vi "Traverse_Space_Server.vi"(6 "Probe Support":T1=[{"Max"=15.0, "Min"=-15.0}, {"Max"=250.0, "Min"=0.0}, {"Max"=15.0, "Min"=-15.0}] {"Min" format="%#.1f"; "Max" format="%#.1f"}, 7 "Mode":T4(ring), 8 "Traverse Limits":T1=[{"Max"=15001.0, "Min"=12000.0}, {"Max"=1000.0, "Min"=-1000.0}, {"Max"=700.0, "Min"=0.0}] {"Min" format="%#.1f"; "Max" format="%#.1f"}, 9 "Probe Volume":T1=[{"Max"=0.0, "Min"=0.0}, {"Max"=250.0, "Min"=0.0}, {"Max"=15.0, "Min"=-15.0}] {"Min" format="%#.1f"; "Max" format="%#.1f"}, 10 "Exclude Array":T2[](array[typedef]) {"Sizes"."Min" format="%#.1f"; "Sizes"."Max" format="%#.1f"}, 11 "Traverse Name":string) -> (0 "Traverse Limits Out":T1=[{"Max"=15001.0, "Min"=12000.0}, {"Max"=1000.0, "Min"=-1000.0}, {"Max"=700.0, "Min"=0.0}] {"Min" format="%#.1f"; "Max" format="%#.1f"}, 1 "Probe Volume Out":T1=[{"Max"=15.0, "Min"=-15.0}, {"Max"=250.0, "Min"=0.0}, {"Max"=15.0, "Min"=-15.0}] {"Min" format="%#.1f"; "Max" format="%#.1f"}, 2 "Exclude Array Out":T2[](array[typedef])=[{"Sizes"=[{"Max"=15000.0, "Min"=0.0}, {"Max"=1000.0, "Min"=-1000.0}, {"Max"=300.0, "Min"=0.0}], "Name"="Roughness Elements", "Exclude Type"=enum."Allow only vertical moves"}, {"Sizes"=[{"Max"=17000.0, "Min"=16000.0}, {"Max"=200.0, "Min"=-200.0}, {"Max"=-50.0, "Min"=-250.0}], "Name"="B204", "Exclude Type"=enum."Exclude completely"}] {"Sizes"."Min" format="%#.1f"; "Sizes"."Max" format="%#.1f"}, 3 "Error Comments":string, 4 "Probe Support Out":T1=[{"Max"=15.0, "Min"=-15.0}, {"Max"=250.0, "Min"=0.0}, {"Max"=15.0, "Min"=-15.0}] {"Min" format="%#.1f"; "Max" format="%#.1f"}, 5 "Space File":path)   [LabVIEW 2014]
uses:
  Gen Trav/Route mapping/Exclude_cluster.ctl
  Gen Trav/Route mapping/Box_size.ctl
  Gen Trav/Route mapping/Exclusion_type.ctl
  Globals/Constants_global.vi
panel:
  # "(Relative to measurement position)"
  # "X                           Y                          Z"
  # "(Relative to measurement position)"
  # "X                           Y                          Z"
  # "X                           Y                          Z"
  # "X                           Y                          Z"
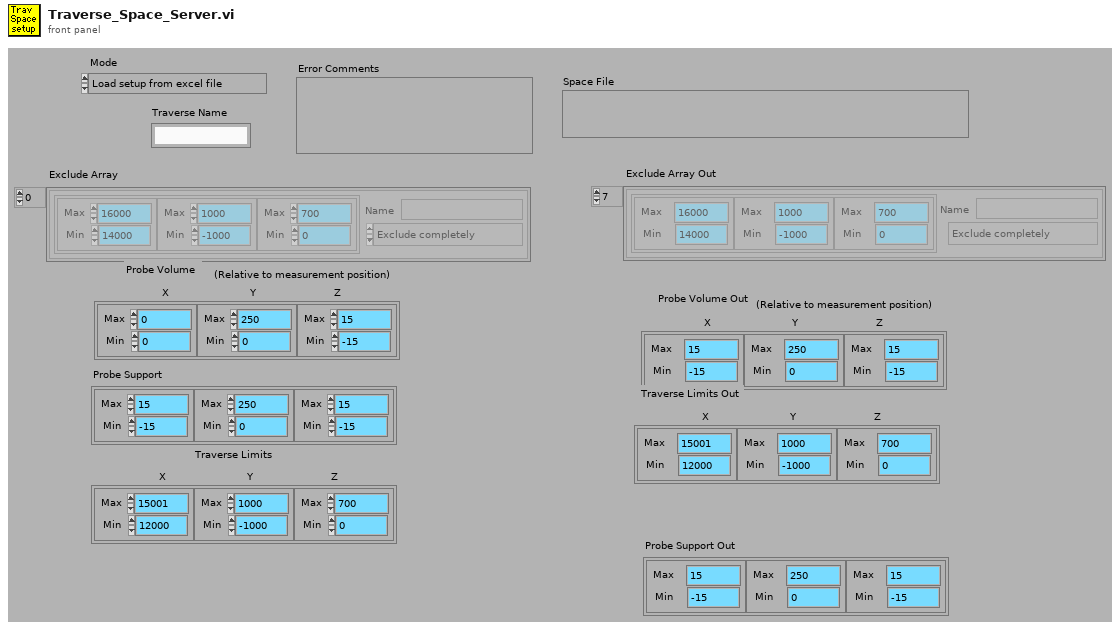
[diagram p1: front panel]
types:
  T1 = typedef "Box_size.ctl" = cluster{"Max":sgl, "Min":sgl}[]
  T2 = typedef "Exclude_cluster.ctl" = cluster{"Sizes":T1, "Name":string, "Exclude Type":T3}
  T3 = typedef "Exclusion_type.ctl" = enum16{"Exclude completely", "Allow only vertical moves"}
  T4 = enum16{"Load setup from excel file", "Save setup to excel file"}
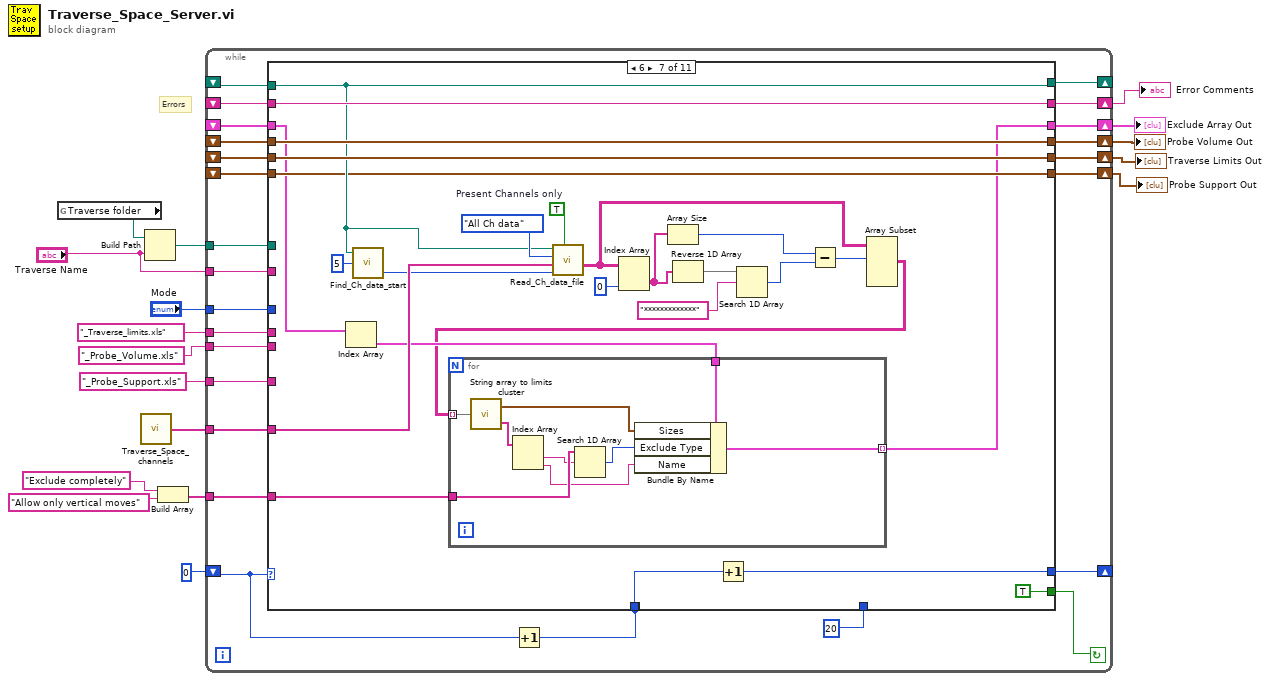
[diagram p0: block diagram]
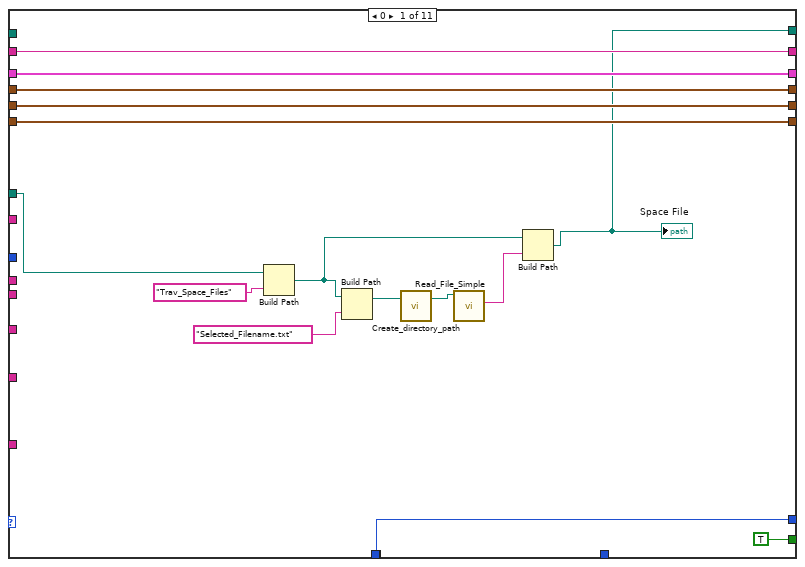
[diagram p2: hidden frame]
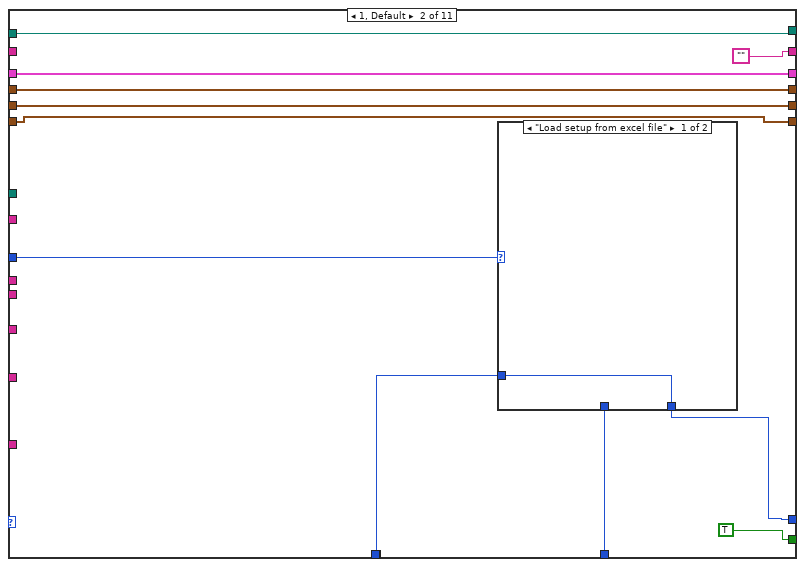
[diagram p3: hidden frame]
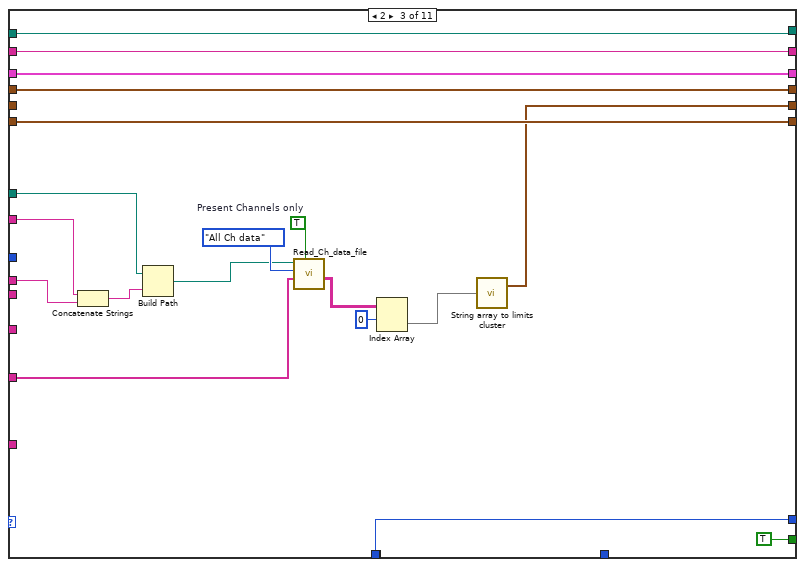
[diagram p5: hidden frame]
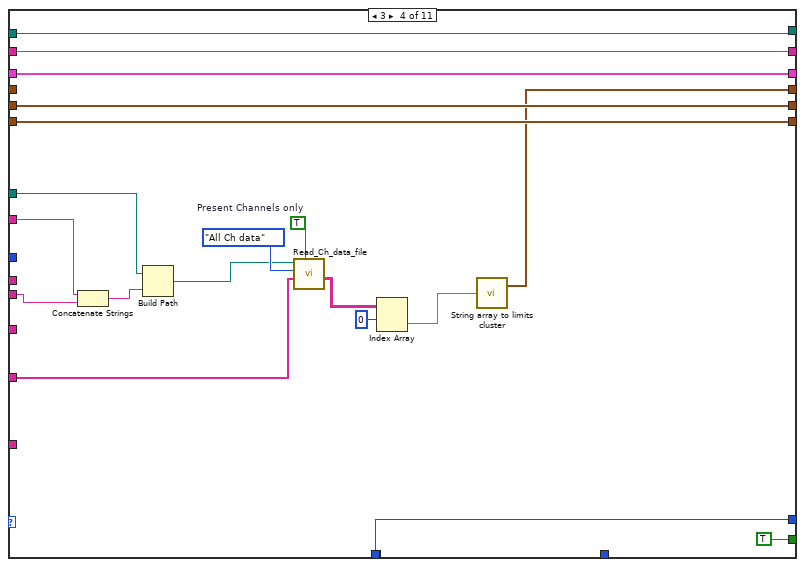
[diagram p6: hidden frame]
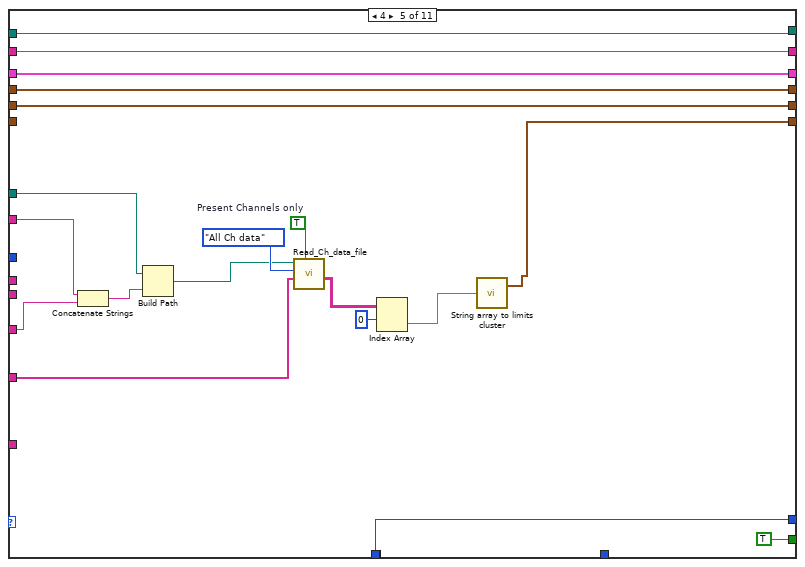
[diagram p7: hidden frame]
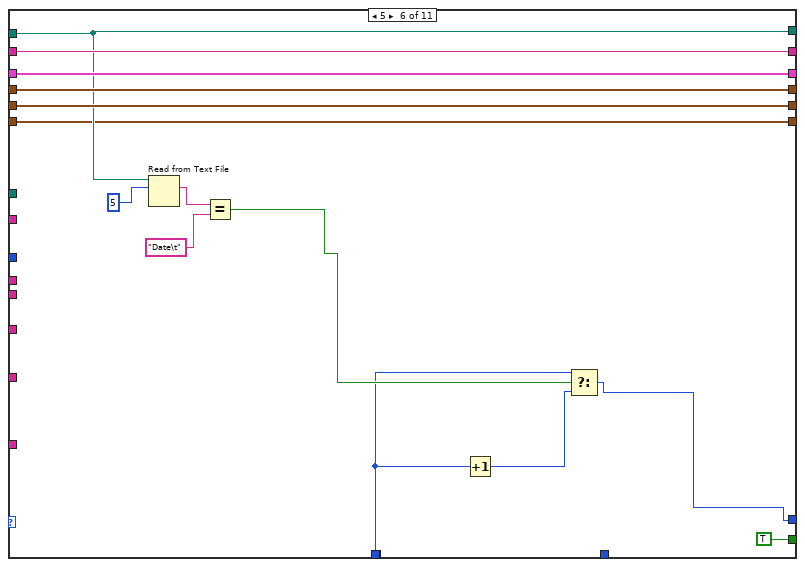
[diagram p8: hidden frame]
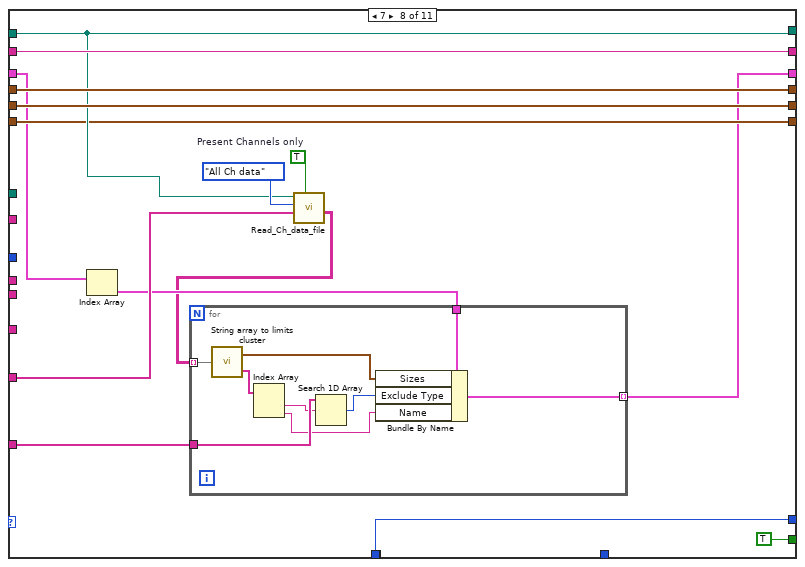
[diagram p9: hidden frame]
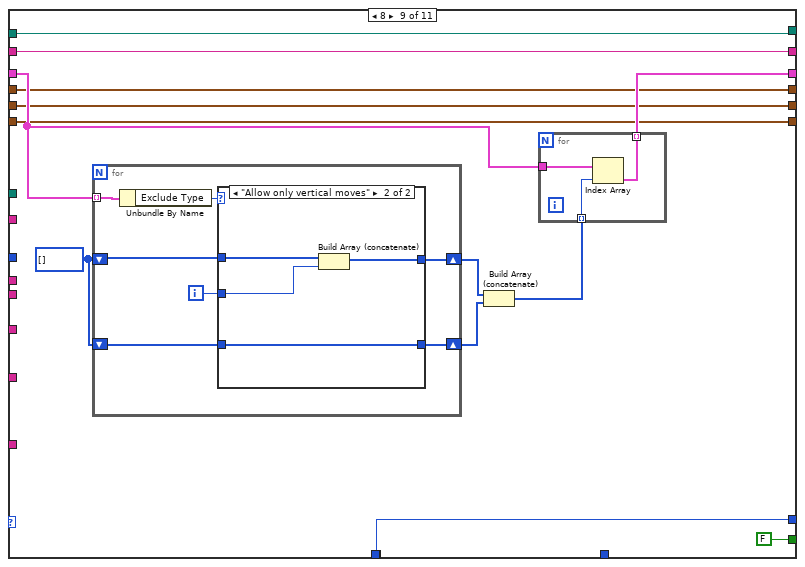
[diagram p10: hidden frame]
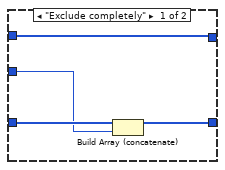
[diagram p11: hidden frame]
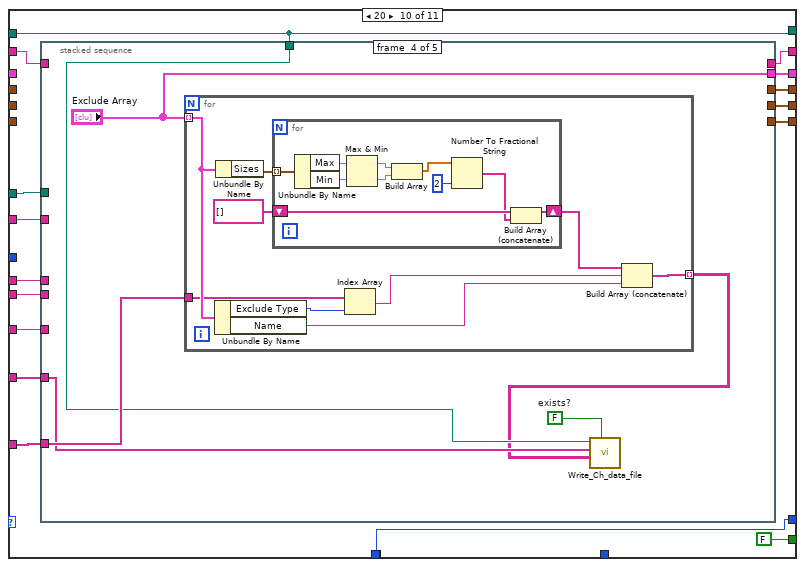
[diagram p12: hidden frame]
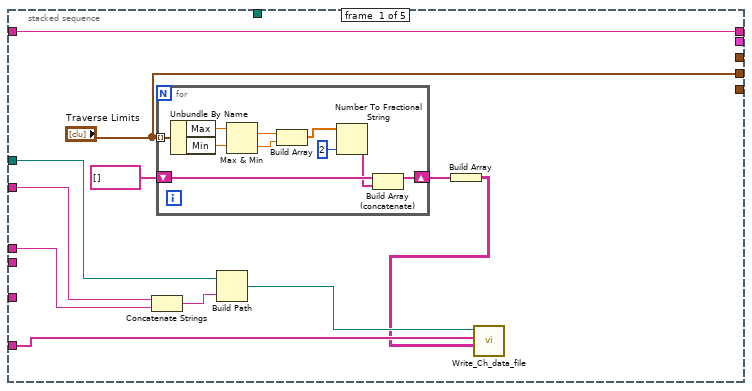
[diagram p13: hidden frame]
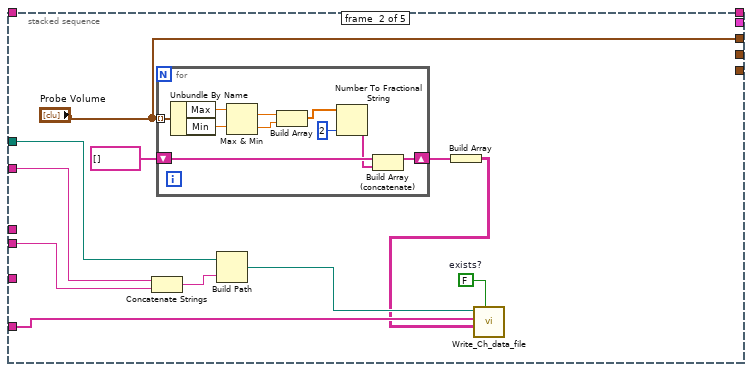
[diagram p14: hidden frame]
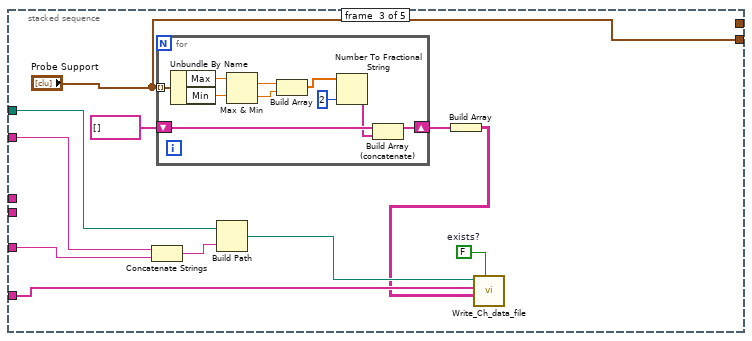
[diagram p15: hidden frame]
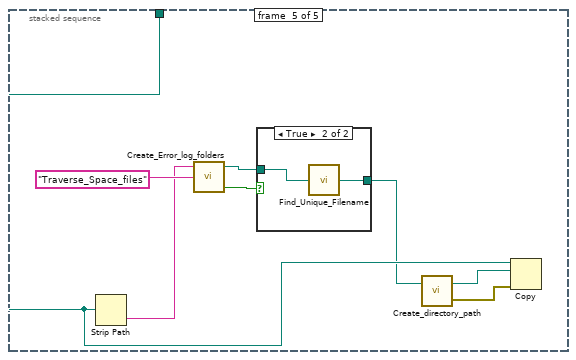
[diagram p16: hidden frame]
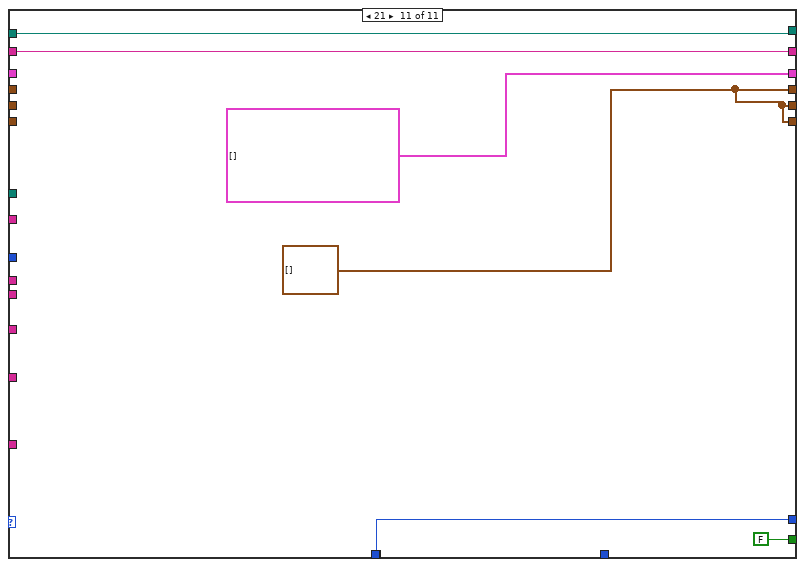
[diagram p18: hidden frame]
diagram:
  # "Errors"
  n1 = global read "Constants_global.vi" "Traverse folder"() -> (w6:path)
  n2 = call "Traverse_Space_channels.vi"() -> ("Channel Names"=w7:string[])
  n3 = Build Path(base path=w6, name or relative path="Traverse Name") -> (appended path=w5:path)
  n4 = Build Array("Exclude completely", "Allow only vertical moves") -> (w11:string[])
  n5 = while {
    tunnel: w11 -> [w29]
    shift-left: _ -> [w32]
    shift-right: [w31] -> w10
    tunnel: "Mode" -> [w39]
    shift-left: _ -> [w35]
    shift-right: [w34] -> w15
    shift-left: _ -> [w37]
    shift-right: [w36] -> w9
    shift-left: _ -> [w38]
    shift-right: [w28] -> w16
    shift-left: 0 -> [w41]
    shift-right: [w40] -> _
    shift-right: [w27] -> w8
    shift-left: _ -> [w26]
    shift-right: [w25] -> _
    shift-left: _ -> [w24]
    tunnel: w7 -> [w23]
    tunnel: w5 -> [w22]
    tunnel: "Traverse Name" -> [w21]
    tunnel: "_Traverse_limits.xls" ("string") -> [w20]
    tunnel: "_Probe_Volume.xls" ("string") -> [w19]
    tunnel: "_Probe_Support.xls" ("string") -> [w18]
    stop <- w42 continue-if-true
    n6 = Increment(x=w41) -> (x+1=w30:i32)
    n7 = case shown="6" w41 {
      tunnel: [TRUE TRUE TRUE TRUE TRUE TRUE TRUE TRUE FALSE FALSE FALSE] -> w42
      tunnel: w30 -> [w53 w64 _ _ _ _ _ _ w211 w240 w352]
      tunnel: [w53 w62 w85 w105 w125 w129 w142 w190 w211 w240 w352] -> w40
      tunnel: w39 -> [_ w68 _ _ _ _ _ _ _ _ _]
      tunnel: w38 -> [w56 w67 w73 w94 w114 w140 w144 w179 w206 _ _]
      tunnel: w37 -> [w55 w66 w89 _ w109 w137 w160 w184 w203 _ _]
      tunnel: [w55 w66 w89 w90 w109 w137 w160 w184 w203 w242 w348] -> w36
      tunnel: w35 -> [w54 w65 _ w91 w112 w138 w161 w185 w202 _ _]
      tunnel: [w54 w65 w71 w91 w112 w138 w161 w185 w202 w241 w348] -> w34
      tunnel: 20 -> [_ w63 _ _ _ _ _ _ _ _ _]
      tunnel: w32 -> [w57 _ w72 w93 w113 w139 w162 w186 w212 w244 w349]
      tunnel: [w57 "" w72 w93 w113 w139 w162 w186 w212 w245 w349] -> w31
      tunnel: w30 -> [_ _ w85 w105 w125 w131 w166 w190 _ _ _]
      tunnel: w29 -> [_ _ _ _ _ _ w147 w181 _ w246 _]
      tunnel: [w56 w67 w73 w94 w114 w140 w143 w178 w205 w243 T2[] [] ("Exclude Array")] -> w28
      tunnel: [w51 w61 w87 w107 w110 w128 w156 w182 w201 w239 w348] -> w27
      tunnel: w26 -> [w51 w61 w87 w107 _ w128 w156 w182 w201 _ _]
      tunnel: [w44 w60 w86 w106 w126 w136 w157 w183 w204 w238 w347] -> w25
      tunnel: w24 -> [_ w60 w86 w106 w126 w136 w157 w183 w204 w238 w347]
      tunnel: w23 -> [_ _ w78 w99 w119 _ w163 w187 _ w234 _]
      tunnel: w22 -> [w43 _ w81 w101 w121 _ _ _ _ w237 _]
      tunnel: w21 -> [_ _ w80 w100 w120 _ _ _ _ w236 _]
      tunnel: w20 -> [_ _ w79 _ _ _ _ _ _ w235 _]
      tunnel: w19 -> [_ _ _ w92 _ _ _ _ _ w233 _]
      tunnel: w18 -> [_ _ _ _ w111 _ _ _ _ w232 _]
      frame 0 {
        n8 = Build Path(base path=w43, name or relative path="Trav_Space_Files" ("Substring")) -> (appended path=w46:path)
        n9 = Build Path(base path=w46, name or relative path="Selected_Filename.txt" ("Substring")) -> (appended path=w50:path)
        n10 = call "Create_directory_path.vi"("Path name"=w50) -> ("Path name Out"=w49:path)  [unwired: 1 in, 1 out]
        n11 = call "Read_File_Simple.vi"("Filename"=w49) -> ("string"=w45:string)  [unwired: 2 in, 7 out]
        n12 = Build Path(base path=w46, name or relative path=w45) -> (appended path=w44:path)
        "Space File" <- w44
      }
      frame 1, Default {
        n13 = case shown="\"Load setup from excel file\"" w68 {
          tunnel: w64 -> [w69 _]
          tunnel: [w69 w70] -> w62
          tunnel: w63 -> [_ w70]
          frame "Load setup from excel file" {
          }
          frame "Save setup to excel file" {
          }
        }
      }
      frame 2 {
        w83 = TRUE  # Present Channels only
        n14 = Concatenate Strings(w80, w79) -> (w82:string)
        n15 = Build Path(base path=w81, name or relative path=w82) -> (appended path=w77:path)
        n16 = call "Read_Ch_data_file.vi"("Present Channels only"=w83, "Present Channels"=w78, "Output"=enum16{"All Ch data", "The last few rows"}."All Ch data", "Filename"=w77) -> ("Channel Values"=w76:string[][])  [unwired: 1 in, 4 out]
        n17 = Index Array(array=w76, index (row)=0) -> (element=w74:string[])  [unwired: 1 in]
        n18 = call "String array to limits cluster.vi"("Channel Values in"=w74) -> ("Limits out"=w71:T1)  [unwired: 1 out]
      }
      frame 3 {
        w103 = TRUE  # Present Channels only
        n19 = Concatenate Strings(w100, w92) -> (w102:string)
        n20 = Build Path(base path=w101, name or relative path=w102) -> (appended path=w98:path)
        n21 = call "Read_Ch_data_file.vi"("Present Channels only"=w103, "Present Channels"=w99, "Output"=enum16{"All Ch data", "The last few rows"}."All Ch data", "Filename"=w98) -> ("Channel Values"=w97:string[][])  [unwired: 1 in, 4 out]
        n22 = Index Array(array=w97, index (row)=0) -> (element=w95:string[])  [unwired: 1 in]
        n23 = call "String array to limits cluster.vi"("Channel Values in"=w95) -> ("Limits out"=w90:T1)  [unwired: 1 out]
      }
      frame 4 {
        w123 = TRUE  # Present Channels only
        n24 = Concatenate Strings(w120, w111) -> (w122:string)
        n25 = Build Path(base path=w121, name or relative path=w122) -> (appended path=w118:path)
        n26 = call "Read_Ch_data_file.vi"("Present Channels only"=w123, "Present Channels"=w119, "Output"=enum16{"All Ch data", "The last few rows"}."All Ch data", "Filename"=w118) -> ("Channel Values"=w117:string[][])  [unwired: 1 in, 4 out]
        n27 = Index Array(array=w117, index (row)=0) -> (element=w115:string[])  [unwired: 1 in]
        n28 = call "String array to limits cluster.vi"("Channel Values in"=w115) -> ("Limits out"=w110:T1)  [unwired: 1 out]
      }
      frame 5 {
        n29 = Read from Text File(file (use dialog)=w136, count=5) -> (text=w134:string)  [unwired: 2 in, 3 out]
        n30 = Equal?(x=w134, y="Date\t") -> (x = y?=w132:bool)
        n31 = Increment(x=w131) -> (x+1=w130:i32)
        n32 = Select(t=w131, s=w132, f=w130) -> (s? t:f=w129:i32)
      }
      frame 6 {
        w164 = TRUE  # Present Channels only
        n33 = Index Array(array=w144) -> (element=w146:T2)  [unwired: 1 in]
        n34 = call "Find_Ch_data_start.vi"("Approx No Of Columns"=5, "Filename"=w157) -> ("Start of read offset output"=w158:i32)  [unwired: 1 in, 2 out]
        n35 = call "Read_Ch_data_file.vi"("Present Channels only"=w164, "Start of read offset (chars.: 0)"=w158, "Present Channels"=w163, "Output"=enum16{"All Ch data", "The last few rows"}."All Ch data", "Filename"=w157) -> ("Channel Values"=w149:string[][])  [unwired: 4 out]
        n36 = Index Array(array=w149, index (col)=0 ("index (row)")) -> (element=w152:string[])  [unwired: 1 in]
        n37 = Array Size(array=w152) -> (size(s)=w151:i32)
        n38 = Reverse 1D Array(array=w152) -> (reversed array=w154:string[])
        n39 = Increment(x=w166) -> (x+1=w142:i32)
        n40 = Search 1D Array(1D array=w154, element="*************") -> (index of element=w150:i32)  [unwired: 1 in]
        n41 = Subtract(x=w151, y=w150) -> (x-y=w148:i32)
        n42 = Array Subset(array=w149, index (row)=w148) -> (w145:string[][])  [unwired: 3 in]
        n43 = for {
          tunnel: w147 -> [w175]
          tunnel: w146 -> [w173]
          tunnel: w145 -> [w169] mode=indexing
          tunnel: [w168] -> w143 mode=indexing
          n44 = call "String array to limits cluster.vi"("Channel Values in"=w169) -> ("Limits out"=w172:T1, "Channel Values out"=w176:string[])
          n45 = Index Array(array=w176) -> (element #1=w174:string, element #2=w171:string)  [unwired: 2 in]
          n46 = Search 1D Array(1D array=w175, element=w174) -> (index of element=w170:i32)  [unwired: 1 out]
          n47 = Bundle By Name(cluster=w173, "Sizes"=w172, "Exclude Type"=w170, "Name"=w171) -> (w168:T2)
        }
      }
      frame 7 {
        w188 = TRUE  # Present Channels only
        n48 = Index Array(array=w179) -> (element=w180:T2)  [unwired: 1 in]
        n49 = call "Read_Ch_data_file.vi"("Present Channels only"=w188, "Present Channels"=w187, "Output"=enum16{"All Ch data", "The last few rows"}."All Ch data", "Filename"=w183) -> ("Channel Values"=w177:string[][])  [unwired: 1 in, 4 out]
        n50 = for {
          tunnel: w181 -> [w199]
          tunnel: w180 -> [w197]
          tunnel: w177 -> [w193] mode=indexing
          tunnel: [w192] -> w178 mode=indexing
          n51 = call "String array to limits cluster.vi"("Channel Values in"=w193) -> ("Limits out"=w196:T1, "Channel Values out"=w200:string[])
          n52 = Index Array(array=w200) -> (element #1=w198:string, element #2=w195:string)  [unwired: 2 in]
          n53 = Search 1D Array(1D array=w199, element=w198) -> (index of element=w194:i32)  [unwired: 1 out]
          n54 = Bundle By Name(cluster=w197, "Sizes"=w196, "Exclude Type"=w194, "Name"=w195) -> (w192:T2)
        }
      }
      frame 8 {
        w210 = i32[] []
        n55 = for {
          tunnel: w206 -> [w217] mode=indexing
          shift-right: [w221] -> w208
          shift-left: w210 -> [w222]
          shift-right: [w220] -> w209
          shift-left: w210 -> [w219]
          i -> [w218]
          n56 = Unbundle By Name(w217) -> ("Exclude Type"=w223:T3)
          n57 = case shown="\"Allow only vertical moves\"" w223 {
            tunnel: w222 -> [w225 w231]
            tunnel: [w225 w230] -> w221
            tunnel: [w226 w229] -> w220
            tunnel: w219 -> [w227 w229]
            tunnel: w218 -> [w224 w228]
            frame "Exclude completely" {
              n58 = Build Array (concatenate)(w227, w224) -> (w226:i32[])
            }
            frame "Allow only vertical moves" {
              n59 = Build Array (concatenate)(w231, w228) -> (w230:i32[])
            }
          }
        }
        n60 = Build Array (concatenate)(w208, w209) -> (w207:i32[])
        n61 = for {
          tunnel: w207 -> [w216] mode=indexing
          tunnel: w206 -> [w215]
          tunnel: [w214] -> w205 mode=indexing
          n62 = Index Array(array=w215, index=w216) -> (element=w214:T2)
        }
      }
      frame 20 {
        n63 = stacked-sequence {
          tunnel: w246 -> [_ _ _ w316 _]
          tunnel: [w248 _ _ _ _] -> w245
          tunnel: w244 -> [w248 _ _ _ _]
          tunnel: [_ _ _ "Exclude Array" _] -> w243
          tunnel: [_ "Probe Volume" _ _ _] -> w242
          tunnel: ["Traverse Limits" _ _ _ _] -> w241
          tunnel: w238 -> [_ _ _ w314 w340]
          tunnel: [_ _ "Probe Support" _ _] -> w239
          tunnel: w237 -> [w256 w278 w299 _ _]
          tunnel: w236 -> [w255 w277 w298 _ _]
          tunnel: w235 -> [w253 _ _ _ _]
          tunnel: w234 -> [w251 w274 w295 w313 _]
          tunnel: w233 -> [_ w270 _ _ _]
          tunnel: w232 -> [_ _ w291 _ _]
          frame #0 {
            n64 = Concatenate Strings(w255, w253) -> (w254:string)
            n65 = for {
              shift-right: [w264] -> w250
              shift-left: string[] [] -> [w266]
              tunnel: "Traverse Limits" -> [w261] mode=indexing
              n66 = Unbundle By Name(w261) -> ("Max"=w260:sgl, "Min"=w259:sgl)
              n67 = Max & Min(x=w260, y=w259) -> (max(x,y)=w263:sgl, min(x,y)=w262:sgl)
              n68 = Build Array(w263, w262) -> (w268:sgl[])
              n69 = Number To Fractional String(number=w268, precision (6)=i16 2) -> (F-format string=w265:string[])  [unwired: 2 out]
              n70 = Build Array (concatenate)(w266, w265) -> (w264:string[])
            }
            n71 = Build Path(base path=w256, name or relative path=w254) -> (appended path=w252:path)
            n72 = Build Array(w250) -> (w249:string[][])
            n73 = call "Write_Ch_data_file.vi"("Channel Values"=w249, "Channel names"=w251, "Filename"=w252) -> ()  [unwired: 4 in, 5 out]
          }
          frame #1 {
            w269 = FALSE  # exists?
            n74 = Concatenate Strings(w277, w270) -> (w276:string)
            n75 = for {
              shift-right: [w285] -> w273
              shift-left: string[] [] -> [w287]
              tunnel: "Probe Volume" -> [w282] mode=indexing
              n76 = Unbundle By Name(w282) -> ("Max"=w281:sgl, "Min"=w280:sgl)
              n77 = Max & Min(x=w281, y=w280) -> (max(x,y)=w284:sgl, min(x,y)=w283:sgl)
              n78 = Build Array(w284, w283) -> (w289:sgl[])
              n79 = Number To Fractional String(number=w289, precision (6)=i16 2) -> (F-format string=w286:string[])  [unwired: 2 out]
              n80 = Build Array (concatenate)(w287, w286) -> (w285:string[])
            }
            n81 = Build Path(base path=w278, name or relative path=w276) -> (appended path=w275:path)
            n82 = Build Array(w273) -> (w272:string[][])
            n83 = call "Write_Ch_data_file.vi"("exists?"=w269, "Channel Values"=w272, "Channel names"=w274, "Filename"=w275) -> ()  [unwired: 3 in, 5 out]
          }
          frame #2 {
            w290 = FALSE  # exists?
            n84 = Concatenate Strings(w298, w291) -> (w297:string)
            n85 = for {
              shift-right: [w306] -> w294
              shift-left: string[] [] -> [w308]
              tunnel: "Probe Support" -> [w303] mode=indexing
              n86 = Unbundle By Name(w303) -> ("Max"=w302:sgl, "Min"=w301:sgl)
              n87 = Max & Min(x=w302, y=w301) -> (max(x,y)=w305:sgl, min(x,y)=w304:sgl)
              n88 = Build Array(w305, w304) -> (w310:sgl[])
              n89 = Number To Fractional String(number=w310, precision (6)=i16 2) -> (F-format string=w307:string[])  [unwired: 2 out]
              n90 = Build Array (concatenate)(w308, w307) -> (w306:string[])
            }
            n91 = Build Path(base path=w299, name or relative path=w297) -> (appended path=w296:path)
            n92 = Build Array(w294) -> (w293:string[][])
            n93 = call "Write_Ch_data_file.vi"("exists?"=w290, "Channel Values"=w293, "Channel names"=w295, "Filename"=w296) -> ()  [unwired: 3 in, 5 out]
          }
          frame #3 {
            w311 = FALSE  # exists?
            n94 = for {
              tunnel: "Exclude Array" -> [w323] mode=indexing
              tunnel: w316 -> [w321]
              tunnel: [w317] -> w312 mode=indexing
              n95 = Unbundle By Name(w323) -> ("Exclude Type"=w322:T3, "Name"=w318:string)
              n96 = Unbundle By Name(w323) -> ("Sizes"=w325:T1)
              n97 = for {
                tunnel: w325 -> [w335] mode=indexing
                shift-right: [w330] -> w320
                shift-left: string[] [] -> [w332]
                n98 = Unbundle By Name(w335) -> ("Max"=w329:sgl, "Min"=w328:sgl)
                n99 = Max & Min(x=w329, y=w328) -> (max(x,y)=w327:sgl, min(x,y)=w326:sgl)
                n100 = Build Array(w327, w326) -> (w334:sgl[])
                n101 = Number To Fractional String(number=w334, precision (6)=i16 2) -> (F-format string=w331:string[])  [unwired: 2 out]
                n102 = Build Array (concatenate)(w332, w331) -> (w330:string[])
              }
              n103 = Index Array(array=w321, index=w322) -> (element=w319:string)
              n104 = Build Array (concatenate)(w320, w319, w318) -> (w317:string[])
            }
            n105 = call "Write_Ch_data_file.vi"("exists?"=w311, "Channel Values"=w312, "Channel names"=w313, "Filename"=w314) -> ()  [unwired: 3 in, 5 out]
          }
          frame #4 {
            n106 = Strip Path(path=w340) -> (name=w339:string)  [unwired: 1 out]
            n107 = call "Create_Error_log_folders.vi"("Log Folder"="Traverse_Space_files", "Log Filename"=w339) -> ("exists?"=w342:bool, "Local Log File"=w341:path)  [unwired: 1 in, 1 out]
            n108 = case shown="True" w342 {
              tunnel: [w344 w346] -> w338
              tunnel: w341 -> [w344 w345]
              frame False {
              }
              frame True {
                n109 = call "Find_Unique_Filename.vi"("Path In"=w345) -> ("Unique Path Out"=w346:path)  [unwired: 1 in, 1 out]
              }
            }
            n110 = call "Create_directory_path.vi"("Path name"=w338) -> ("error out"=w336:errorcluster, "Path name Out"=w337:path)  [unwired: 1 in]
            n111 = Copy(8:w336, 10:w337, 11:w340) -> ()  [unwired: 5 out]
          }
        }
      }
      frame 21 {
        w348 = T1 [] ("Probe Volume")
      }
    }
  }
  "Error Comments" <- w10
  "Probe Volume Out" <- w9
  "Traverse Limits Out" <- w15
  "Exclude Array Out" <- w16
  "Probe Support Out" <- w8
